vi "Xctrl interface-Set timeline range.vi"(8 "error in (no error)":errorcluster, 10 "X-axis max/min (across all loaded data types)":cluster{"X-axis max":dbl, "X-axis min":dbl}) -> (0 "error out":errorcluster)   [LabVIEW 2013]
uses:
  XGrapher.xctl
  Global variables/gl_Functional Imaging-Global variables.vi
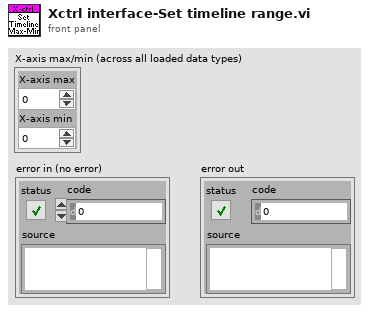
[diagram p1: front panel]
types:
  T1 = typedef "Functional Imging UI Refs.ctl" = cluster{"Menu ref":refnum<k9>, "Image control":refnum<vi>, "VI ref":refnum<vi>, "XGrapher":refnum<vi>, "Smoothing":refnum<vi>, "POI Averaging":refnum<vi>, "Normalize":refnum<vi>, "POI data points in each trial":refnum<vi>, "Channel":refnum<vi>, "Experiment data folder path":refnum<vi>, "[ROI vis]":refnum<vi>, "[Groups] visbl":T2, "Group Name":refnum<vi>, "POI index":refnum<vi>, "Trial No.":refnum<vi>, "Intensity Zoom":refnum<vi>, "Trial Cursor Enabled":refnum<vi>, "Number of Trials (ind 1)":refnum<vi>, "Number of Trials (ind 2)":refnum<vi>, "MiniScans Available":refnum<vi>, "POI Available":refnum<vi>, "Defer graph updates":refnum<vi>, "Waveform selector":refnum<vi>, "#of selected POI":refnum<vi>, "#of selected MiniScans":refnum<vi>, "#of selected groups":refnum<vi>, "Max Z-Projection":refnum<vi>, "Z-Plane Selector":refnum<vi>, "Index of miniscan point to visualise":refnum<vi>, "ROI vis. mode":refnum<vi>, "Total # of points":refnum<vi>, "Index of group clicked on":refnum<vi>, "Pane 1":refnum<vi>, "Pane 2":refnum<vi>, "Pane 3":refnum<vi>, "Pane 4":refnum<vi>, "Pane 5":refnum<vi>, "Pane 6":refnum<vi>, "Deselect all ROI":refnum<vi>, "Deselect all groups":refnum<vi>}
  T2 = typedef "Groups array referecne.ctl" = refnum<vi>
  T3 = typedef "XGrapher.xctl/Xctrl-Timeline graph ref.ctl" = refnum<vi>
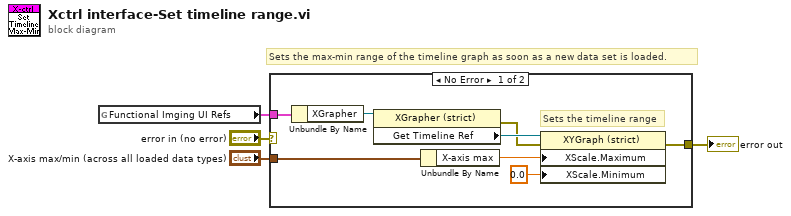
[diagram p0: block diagram]
diagram:
  # "Sets the max-min range of the timeline graph as soon as a new data set is loaded."
  n1 = global read "gl_Functional Imaging-Global variables.vi" "Functional Imging UI Refs"() -> (w1:T1)
  n2 = case shown="No Error" "error in (no error)" {
    selector: "error in (no error)" -> [_ w13]
    tunnel: [w12 w13] -> w4
    tunnel: w1 -> [w11 _]
    tunnel: "X-axis max/min (across all loaded data types)" -> [w10 _]
    frame No Error {
      # "Sets the timeline range"
      n3 = Unbundle By Name(w11) -> ("XGrapher"=w9:refnum<vi>)
      n4 = property on="Property Node" class="XGrapher (strict)"(reference=w9) -> (error out=w7:errorcluster, "Get Timeline Ref"=w8:T3)  [unwired: 1 in, 1 out]
      n5 = Unbundle By Name(w10) -> ("X-axis max"=w6:dbl)
      n6 = property class="XYGraph (strict)"(reference=w8, error in=w7, "XScale.Maximum"=w6, "XScale.Minimum"=0.0 ("X Scale.Range:Minimum")) -> (error out=w12:errorcluster)  [unwired: 1 out]
    }
    frame Error {
    }
  }
  "error out" <- w4
